vi "GHV232 CRAB Receive Data.vi"(0 "VISA resource name":refnum<visa-resource-name>, 11 "error in (no error)":errorcluster) -> (2 "V":bool, 3 "Vmon":dbl format="%#.2g", 4 "VISA resource name 2":refnum<visa-resource-name>, 6 "HV on":bool, 8 "Message":string, 10 "Fault":bool, 13 "I":bool, 14 "Imon":dbl format="%#.2g", 15 "error out":errorcluster)   [LabVIEW 2017]
panel:
  # "This VI decodes the received packet from the power supply.  If the received packet\nis a query response it will update the digital and analog monitors.  An 'Acknowledge \nOK' message is displayed in response to a send command or PS reset command.  If \nit was a version request, the message will give the firmware version.  Otherwise, the \nmessage will give an error response."
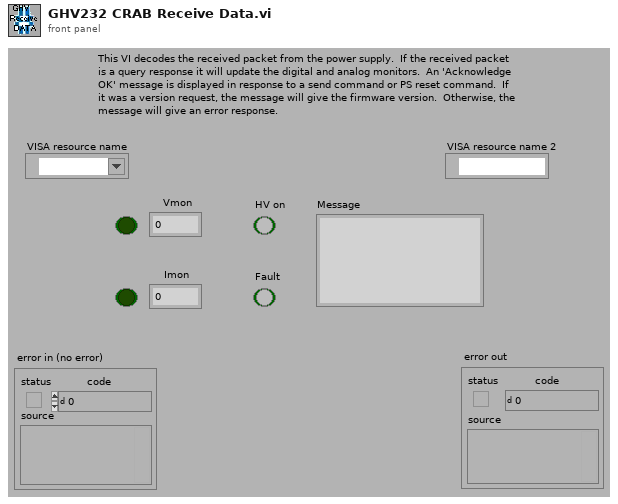
[diagram p1: front panel]
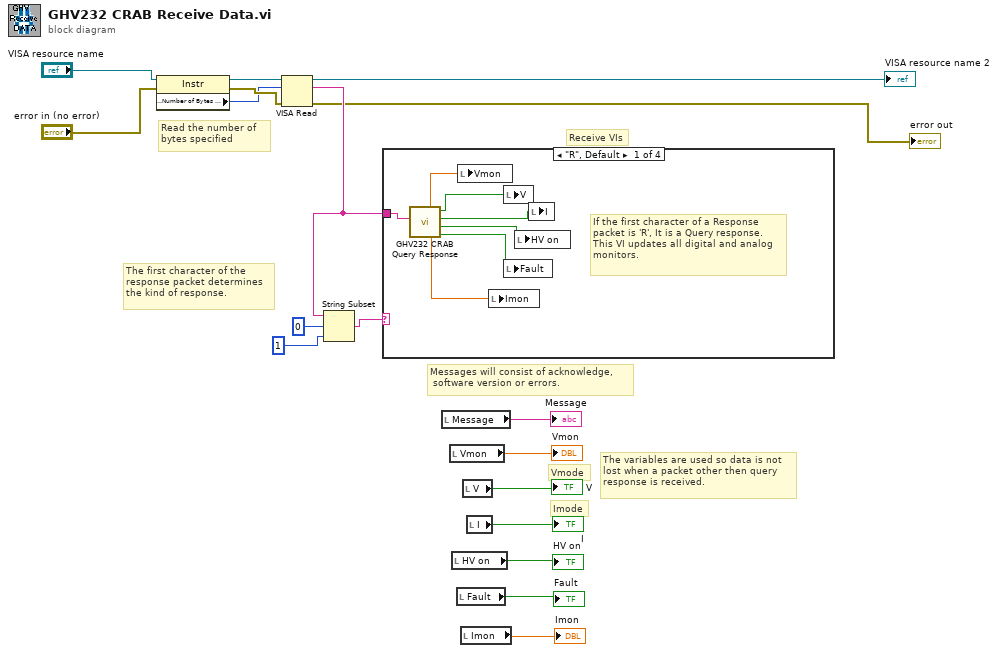
[diagram p0: block diagram]
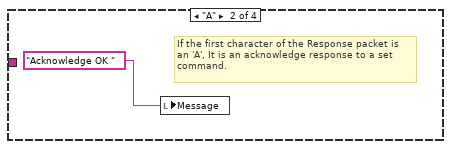
[diagram p2: hidden frame]
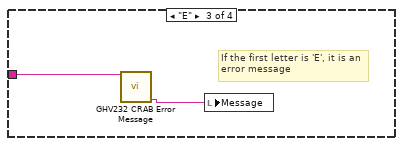
[diagram p3: hidden frame]
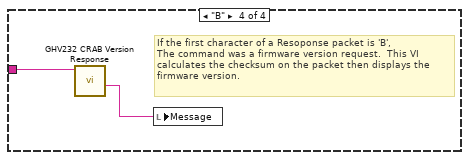
[diagram p4: hidden frame]
diagram:
  # "The variables are used so data is not\nlost when a packet other then query \nresponse is received."
  # "The first character of the\nresponse packet determines\nthe kind of response."
  # "Read the number of \nbytes specified"
  # "Imode"
  # "Vmode"
  # "Receive VIs"
  # "Messages will consist of acknowledge,\n software version or errors."
  n1 = property class="Instr"(reference="VISA resource name", error in="error in (no error)") -> (reference out=w11:refnum<visa-resource-name>, error out=w10:errorcluster, "Serial Settings:Number of Bytes at Serial Port"=w9:u32)
  n2 = VISA Read(VISA resource name=w11, byte count=w9, error in (no error)=w10) -> (VISA resource name out=→"VISA resource name 2":refnum<visa-resource-name>, read buffer=w3:string, error out=→"error out":errorcluster)  [unwired: 1 out]
  n3 = String Subset(string=w3, offset (0)=0, length (rest)=1) -> (substring=w4:string)
  n4 = case shown="\"R\", Default" w4 {
    tunnel: w3 -> [w25 _ w28 w30]
    frame "R", Default {
      # "If the first character of a Response\npacket is 'R', It is a Query response.\nThis VI updates all digital and analog\nmonitors."
      n5 = call "GHV232 CRAB Query Response.vi"("String"=w25) -> ("Fault"=w20:bool, "HV on"=w21:bool, "I mode"=w22:bool, "V mode"=w23:bool, "Current"=w19:dbl, "Voltage"=w24:dbl)  [unwired: 4 in, 1 out]
      n6 = local write "Vmon"(w24) -> ()
      n7 = local write "Imon"(w19) -> ()
      n8 = local write "V"(w23) -> ()
      n9 = local write "Fault"(w20) -> ()
      n10 = local write "HV on"(w21) -> ()
      n11 = local write "I"(w22) -> ()
    }
    frame "A" {
      # "If the first character of the Response packet is\nan 'A', It is an acknowledge response to a set\ncommand."
      n12 = local write "Message"("Acknowledge OK ") -> ()
    }
    frame "E" {
      # "If the first letter is 'E', it is an\nerror message"
      n13 = call "GHV232 CRAB Error Message.vi"("Receive Packet"=w28) -> ("Message"=w27:string)  [unwired: 10 in]
      n14 = local write "Message"(w27) -> ()
    }
    frame "B" {
      # "If the first character of a Resoponse packet is 'B',\nThe command was a firmware version request.  This VI\ncalculates the checksum on the packet then displays the\nfirmware version."
      n15 = call "GHV232 CRAB Version Response.vi"("Recieve Packet"=w30) -> ("Message"=w29:string)  [unwired: 10 in]
      n16 = local write "Message"(w29) -> ()
    }
  }
  n17 = local read "Message"() -> (→"Message":string)
  n18 = local read "Vmon"() -> (→"Vmon":dbl)
  n19 = local read "HV on"() -> (→"HV on":bool)
  n20 = local read "Fault"() -> (→"Fault":bool)
  n21 = local read "Imon"() -> (→"Imon":dbl)
  n22 = local read "V"() -> (→"V":bool)
  n23 = local read "I"() -> (→"I":bool)
